vi "VI Tree.vi"   [LabVIEW 2019]
doc: "This is the instrument driver for the Agilent 8114A. The VI Tree displays all the user-callable VIs of the instrument driver in an organized table."
uses:
  <instrlib>/Pulse Rider PG-1000/Pulse Rider PG-1000.lvlib
panel:
  # "SEE DIAGRAM\nFOR VI TREE."
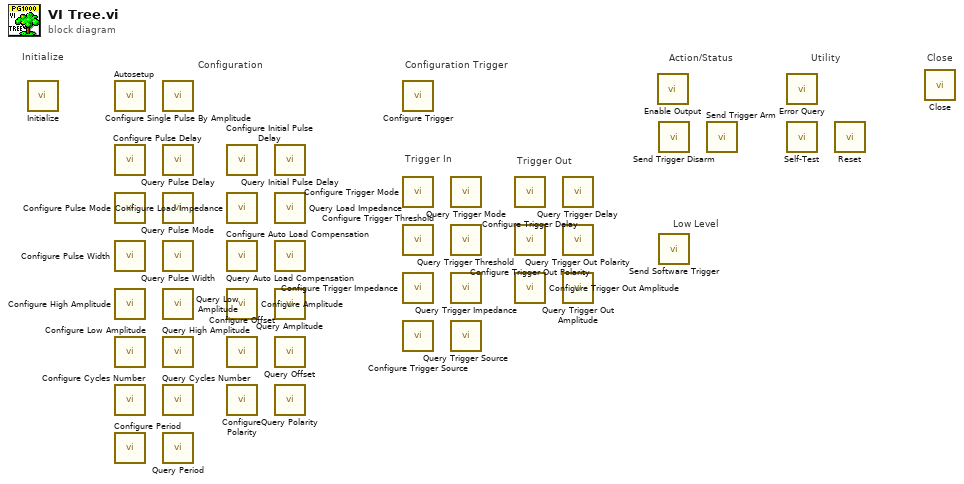
[diagram p0: block diagram]
diagram:
  # "Trigger Out"
  # "Trigger In"
  # "Configuration Trigger"
  # "Low Level"
  # "Configuration"
  # "Utility"
  # "Action/Status"
  # "Close"
  # "Initialize"
  n1 = call <instrlib>:"Initialize.vi"() -> ()  [unwired: 10 in, 2 out]
  n2 = call <instrlib>:"Autosetup.vi"() -> ()  [unwired: 10 in, 2 out]
  n3 = call <instrlib>:"Configure Pulse Delay.vi"() -> ()  [unwired: 10 in, 2 out]
  n4 = call <instrlib>:"Configure Pulse Mode.vi"() -> ()  [unwired: 10 in, 2 out]
  n5 = call <instrlib>:"Configure Pulse Width.vi"() -> ()  [unwired: 10 in, 2 out]
  n6 = call <instrlib>:"Configure High Amplitude.vi"() -> ()  [unwired: 10 in, 2 out]
  n7 = call <instrlib>:"Configure Low Amplitude.vi"() -> ()  [unwired: 10 in, 2 out]
  n8 = call <instrlib>:"Configure Cycles Number.vi"() -> ()  [unwired: 10 in, 2 out]
  n9 = call <instrlib>:"Configure Period.vi"() -> ()  [unwired: 10 in, 2 out]
  n10 = call <instrlib>:"Configure Single Pulse By Amplitude.vi"() -> ()  [unwired: 14 in, 2 out]
  n11 = call <instrlib>:"Query Pulse Delay.vi"() -> ()  [unwired: 9 in, 3 out]
  n12 = call <instrlib>:"Query Pulse Mode.vi"() -> ()  [unwired: 9 in, 3 out]
  n13 = call <instrlib>:"Query Pulse Width.vi"() -> ()  [unwired: 9 in, 3 out]
  n14 = call <instrlib>:"Query Low Amplitude.vi"() -> ()  [unwired: 9 in, 3 out]
  n15 = call <instrlib>:"Query High Amplitude.vi"() -> ()  [unwired: 9 in, 3 out]
  n16 = call <instrlib>:"Query Cycles Number.vi"() -> ()  [unwired: 9 in, 3 out]
  n17 = call <instrlib>:"Query Period.vi"() -> ()  [unwired: 9 in, 3 out]
  n18 = call <instrlib>:"Configure Initial Pulse Delay.vi"() -> ()  [unwired: 10 in, 2 out]
  n19 = call <instrlib>:"Configure Load Impedance.vi"() -> ()  [unwired: 10 in, 2 out]
  n20 = call <instrlib>:"Configure Auto Load Compensation.vi"() -> ()  [unwired: 10 in, 2 out]
  n21 = call <instrlib>:"Configure Amplitude.vi"() -> ()  [unwired: 10 in, 2 out]
  n22 = call <instrlib>:"Configure Offset.vi"() -> ()  [unwired: 10 in, 2 out]
  n23 = call <instrlib>:"Configure Polarity.vi"() -> ()  [unwired: 10 in, 2 out]
  n24 = call <instrlib>:"Query Initial Pulse Delay.vi"() -> ()  [unwired: 9 in, 3 out]
  n25 = call <instrlib>:"Query Load Impedance.vi"() -> ()  [unwired: 9 in, 3 out]
  n26 = call <instrlib>:"Query Auto Load Compensation.vi"() -> ()  [unwired: 9 in, 3 out]
  n27 = call <instrlib>:"Query Amplitude.vi"() -> ()  [unwired: 9 in, 3 out]
  n28 = call <instrlib>:"Query Offset.vi"() -> ()  [unwired: 9 in, 3 out]
  n29 = call <instrlib>:"Query Polarity.vi"() -> ()  [unwired: 9 in, 3 out]
  n30 = call <instrlib>:"Configure Trigger.vi"() -> ()  [unwired: 10 in, 2 out]
  n31 = call <instrlib>:"Configure Trigger Mode.vi"() -> ()  [unwired: 10 in, 2 out]
  n32 = call <instrlib>:"Configure Trigger Threshold.vi"() -> ()  [unwired: 10 in, 2 out]
  n33 = call <instrlib>:"Configure Trigger Impedance.vi"() -> ()  [unwired: 10 in, 2 out]
  n34 = call <instrlib>:"Configure Trigger Source.vi"() -> ()  [unwired: 10 in, 2 out]
  n35 = call <instrlib>:"Query Trigger Mode.vi"() -> ()  [unwired: 9 in, 3 out]
  n36 = call <instrlib>:"Query Trigger Threshold.vi"() -> ()  [unwired: 9 in, 3 out]
  n37 = call <instrlib>:"Query Trigger Impedance.vi"() -> ()  [unwired: 9 in, 3 out]
  n38 = call <instrlib>:"Query Trigger Source.vi"() -> ()  [unwired: 9 in, 3 out]
  n39 = call <instrlib>:"Configure Trigger Delay.vi"() -> ()  [unwired: 10 in, 2 out]
  n40 = call <instrlib>:"Configure Trigger Out Polarity.vi"() -> ()  [unwired: 10 in, 2 out]
  n41 = call <instrlib>:"Configure Trigger Out Amplitude.vi"() -> ()  [unwired: 10 in, 2 out]
  n42 = call <instrlib>:"Query Trigger Delay.vi"() -> ()  [unwired: 9 in, 3 out]
  n43 = call <instrlib>:"Query Trigger Out Polarity.vi"() -> ()  [unwired: 9 in, 3 out]
  n44 = call <instrlib>:"Query Trigger Out Amplitude.vi"() -> ()  [unwired: 9 in, 3 out]
  n45 = call <instrlib>:"Enable Output.vi"() -> ()  [unwired: 10 in, 2 out]
  n46 = call <instrlib>:"Send Trigger Disarm.vi"() -> ()  [unwired: 10 in, 2 out]
  n47 = call <instrlib>:"Send Software Trigger.vi"() -> ()  [unwired: 10 in, 2 out]
  n48 = call <instrlib>:"Send Trigger Arm.vi"() -> ()  [unwired: 10 in, 2 out]
  n49 = call <instrlib>:"Error Query.vi"() -> ()  [unwired: 8 in, 4 out]
  n50 = call <instrlib>:"Self-Test.vi"() -> ()  [unwired: 9 in, 3 out]
  n51 = call <instrlib>:"Reset.vi"() -> ()  [unwired: 10 in, 2 out]
  n52 = call <instrlib>:"Close.vi"() -> ()  [unwired: 11 in, 1 out]
